vi "sio open.vi"(0 "port":i32) -> (5 "port":i32, 8 "Status":i32)   [LabVIEW 2015, in "PCOMM.lvlib"]
doc: "int WINAPI sio_open(int port);"
uses:
  PCOMM.lvlib
  PCOMM.DLL
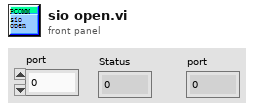
[diagram p1: front panel]
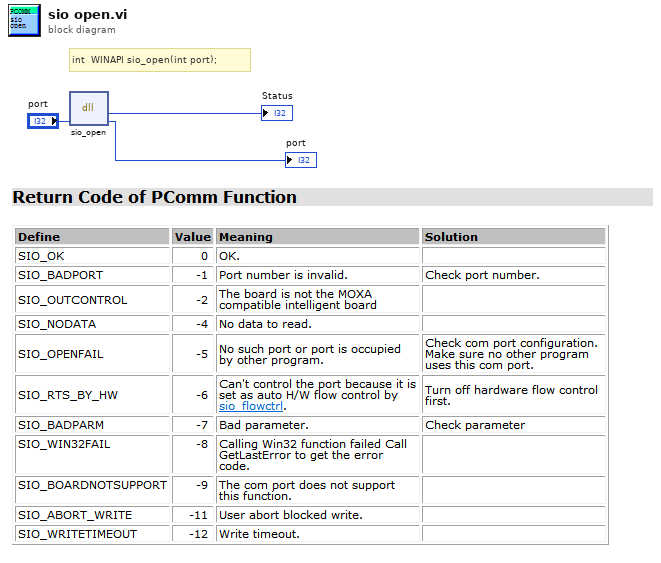
[diagram p0: block diagram]
diagram:
  # "int  WINAPI sio_open(int port);"
  n1 = dll-call lib="PTH2^abs EDesktopLabview串口助手串口助手2.0Ing10_v3.2.0SubVIpcomm库PCOMM.*" fn="sio_open"("port"="port") -> (→"Status":i32, "port"=→"port":i32)  [unwired: 3 in, 2 out]
